vi "2_5.vi"() -> ()   [LabVIEW 2017]
panel:
  out "Number to Array":bool[](array[boolean])
  out "Number":i32
  in  "Array":bool[](array[boolean])
  out "Array OR":bool
  out "Array AND":bool
  out "0, 1":i16
  out "A implies B?":bool
  out "not (A xor B)?":bool
  out "not (A or B)?":bool
  out "A xor B?":bool
  in  "B":bool
  in  "A":bool
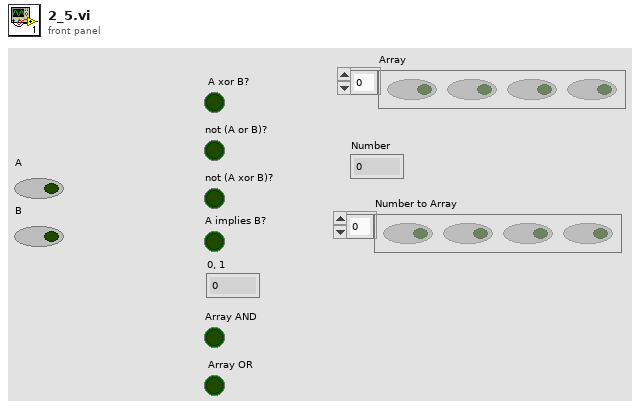
[diagram p1: front panel]
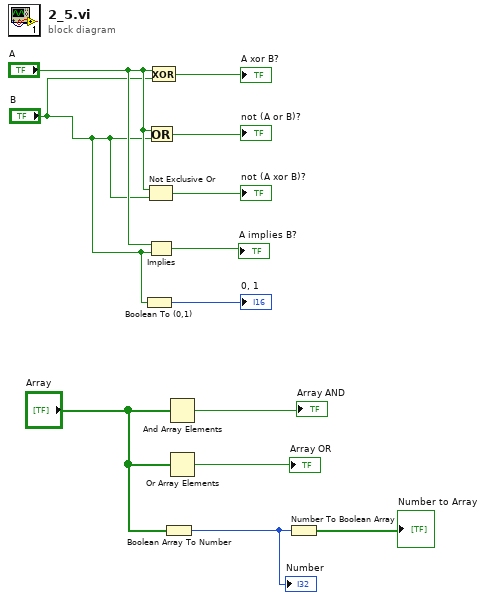
[diagram p0: block diagram]
diagram:
  n1 = Boolean To (0,1)(Boolean="B") -> (0, 1=→"0, 1":i16)
  n2 = Not Exclusive Or(1:"B", 2:"A") -> (0:→"not (A xor B)?":bool)
  n3 = Implies(1:"B", 2:"A") -> (0:→"A implies B?":bool)
  n4 = Or(x="A", y="B") -> (x .or. y?=→"not (A or B)?":bool)
  n5 = Exclusive Or(1:"B", 2:"A") -> (0:→"A xor B?":bool)
  n6 = Boolean Array To Number(Boolean array="Array") -> (number=w2:u32)
  "Number" <- w2
  n7 = And Array Elements(Boolean array="Array") -> (logical AND=→"Array AND":bool)
  n8 = Or Array Elements(Boolean array="Array") -> (logical OR=→"Array OR":bool)
  n9 = Number To Boolean Array(number=w2) -> (Boolean array=→"Number to Array":bool[])
